vi "rp_quickdrop_shortcuts.vi"(10 "FP":string="ac:Array;\nb:Push Button;\nbb:Round LED;\nc:Cluster;\nd:Numeric Control;\ndd:Numeric Indicator;\nen:Enum;\ner:Error In 3D.ctl;\nerr:Error Out 3D.ctl;\np:File Path Control;\npp:File Path Indicator;\ns:String Control;\nss:String Indicator;\nvar:Variant;\nvi:VI Refnum;\nvisa:VISA resource name;", 11 "BD":string="!=:Not Equal?;\n!=0:Not Equal To 0?;\n':Empty String/Path?;\n<:Less?;\n<0:Less Than 0?;\n<=:Less Or Equal?;\n<=0:Less Or Equal To 0?;\n=:Equal?;\n=0:Equal To 0?;\n>:Greater?;\n>0:Greater Than 0?;\n>=:Greater Or Equal?;\n>=0:Greater Or Equal To 0?;\na:Build Array;\naa:Index Array;\nac:Array Constant;\nb:Bundle By Name;\nbb:False Constant;\nbu:Build Path;\nc:Cluster Constant;\ncase:Case Structure;\ndbl:Numeric Constant;\ndia:Diagram Disable Structure;\nf:Format Into String;\nfor:For Loop;\nfs:Flatten To String;\ni:Invoke Node;\nmer:Merge Errors;\nnan:Not A Number/Path/Refnum?;\nop:Open VI Reference;\np:Property Node;\npp:Path Constant;\ns:String Constant;\nsc:Scan From String;\nse:Select;\ntdbl:To Double Precision Float;\ntext:To Extended Precision Float;\nthis:VI Server Reference;\nt1:To Byte Integer;\nt2:To Word Integer;\nt3:To Long Integer;\nt4:To Quad Integer;\ntsgl:To Single Precision Float;\ntt1:To Unsigned Byte Integer;\ntt2:To Unsigned Word Integer;\ntt3:To Unsigned Long Integer;\ntt4:To Unsigned Quad Integer;\nu:Unbundle By Name;\nun:Unflatten From String;\nwh:While Loop;") -> (0 "error out":errorcluster)   [LabVIEW 2019]
doc: "This updates the <b>LABVIEW_DIR\\LabVIEW.ini</b> for rcpacini's Quick Drop Block Diagram and Panel shortcuts.\n\nCreated by: Ryan Pacini"
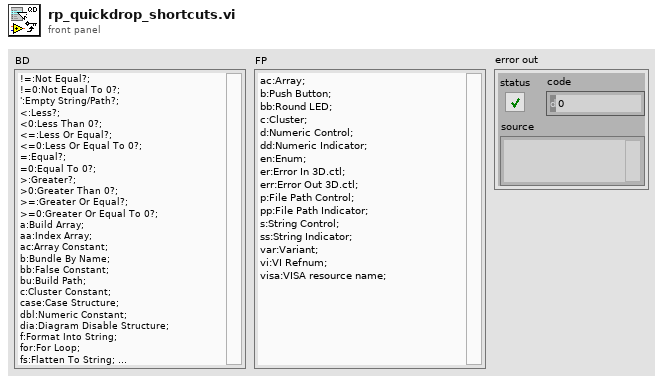
[diagram p1: front panel]
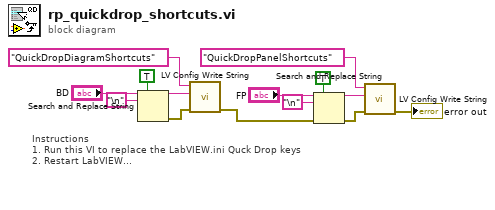
[diagram p0: block diagram]
diagram:
  # "Instructions\n1. Run this VI to replace the LabVIEW.ini Quck Drop keys\n2. Restart LabVIEW..."
  n1 = Search and Replace String(replace all?=TRUE ("replace all? (F)"), input string="BD", search string="\n") -> (result string=w9:string, error out=w8:errorcluster)  [unwired: 5 in, 2 out]
  n2 = call <resource>:"LV Config Write String.vi"("error in (no error)"=w8, "value"=w9, "key"="QuickDropDiagramShortcuts") -> ("error out"=w5:errorcluster)  [unwired: 4 in]
  n3 = Search and Replace String(replace all?=TRUE ("replace all? (F)"), input string="FP", search string="\n", error in=w5) -> (result string=w3:string, error out=w4:errorcluster)  [unwired: 4 in, 2 out]
  n4 = call <resource>:"LV Config Write String.vi"("error in (no error)"=w4, "value"=w3, "key"="QuickDropPanelShortcuts") -> ("error out"=→"error out":errorcluster)  [unwired: 4 in]
